vi "extrnal fgv store.vi"(9 "EMSG_Actions":enum16{"Init", "Set", "Get"}(ring)=enum."Set", 10 "Name":string, 11 "EventMsg in":refnum<class "EventMsg.lvclass">) -> (3 "EventMsg out":refnum<class "EventMsg.lvclass">)   [LabVIEW 2014]
uses:
  Event_class/EventMsg.lvclass
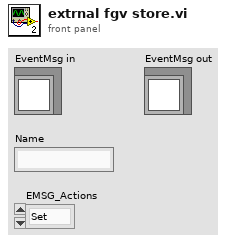
[diagram p1: front panel]
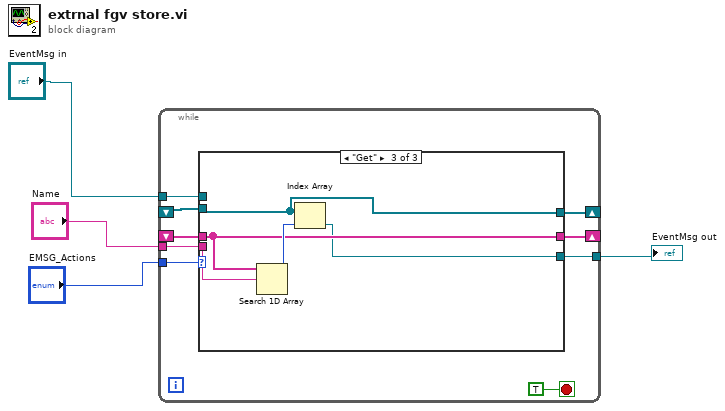
[diagram p0: block diagram]
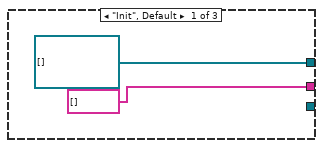
[diagram p2: hidden frame]
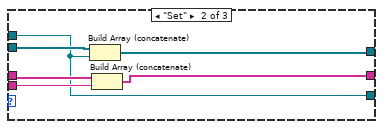
[diagram p3: hidden frame]
diagram:
  n1 = while {
    shift-right: [w11] -> _
    shift-left: _ -> [w9]
    tunnel: "EventMsg in" -> [w10]
    tunnel: "EMSG_Actions" -> [w12]
    shift-right: [w6] -> _
    shift-left: _ -> [w8]
    tunnel: "Name" -> [w7]
    tunnel: [w5] -> w4
    stop <- TRUE stop-if-true
    n2 = case shown="\"Get\"" w12 {
      tunnel: [refnum<class "EventMsg.lvclass">[] [] w20 w23] -> w11
      tunnel: w10 -> [_ w16 _]
      tunnel: w9 -> [_ w21 w23]
      tunnel: w8 -> [_ w19 w24]
      tunnel: w7 -> [_ w18 w26]
      tunnel: [string[] [] w17 w24] -> w6
      tunnel: [_ w16 w22] -> w5
      frame "Init", Default {
      }
      frame "Set" {
        n3 = Build Array (concatenate)(w21, w16) -> (w20:refnum<class "EventMsg.lvclass">[])
        n4 = Build Array (concatenate)(w19, w18) -> (w17:string[])
      }
      frame "Get" {
        n5 = Search 1D Array(1D array=w24, element=w26) -> (index of element=w25:i32)  [unwired: 1 in]
        n6 = Index Array(array=w23, index=w25) -> (element=w22:refnum<class "EventMsg.lvclass">)
      }
    }
  }
  "EventMsg out" <- w4
